vi "Create move.vi"(9 "Destination":T1={"File"=enum."d", "Rank"=enum."4"}, 10 "Source":T1={"File"=enum."d", "Rank"=enum."4"}, 11 "Piece":refnum<class "Piece.lvclass">) -> (3 "Move out":refnum<class "Move.lvclass">)   [LabVIEW 2015, in "Chesslib.lvlib" / "Move.lvclass"]
uses:
  Move.lvclass
  typedef/Square.ctl
  typedef/File.ctl
  typedef/Rank.ctl
  Pieces/Piece/Piece.lvclass
  Chesslib.lvlib
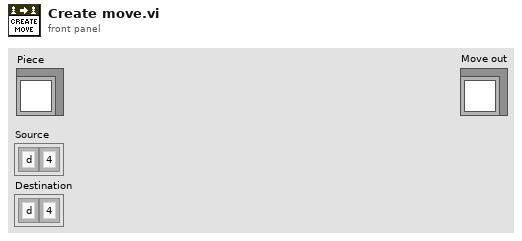
[diagram p1: front panel]
types:
  T1 = typedef "Chesslib.lvlib/Square.ctl" = cluster{"File":T2, "Rank":T3}
  T2 = typedef "Chesslib.lvlib/File.ctl" = enum8{"a", "b", "c", "d", "e", "f", "g", "h"}
  T3 = typedef "Chesslib.lvlib/Rank.ctl" = enum8{"1", "2", "3", "4", "5", "6", "7", "8"}
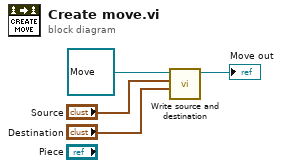
[diagram p0: block diagram]
diagram:
  n1 = call "Write source and destination.vi"("Destination"="Destination", "Source"="Source", "Move in"=refnum<class "Move.lvclass"> refnum) -> ("Move out"=→"Move out":refnum<class "Move.lvclass">)  [unwired: 8 in]
